vi "Example Threshold - CurrentReached Callback.vi"(4 "CurrentReached":refnum<user-event>, 5 "Event Data":T1, 6 "Control Ref":refnum<k24>, 7 "Event Common Data":T2) -> ()   [LabVIEW 2010]
uses:
  C:/tf/play/labview/Tinkerforge.dll
  Tinkerforge.dll
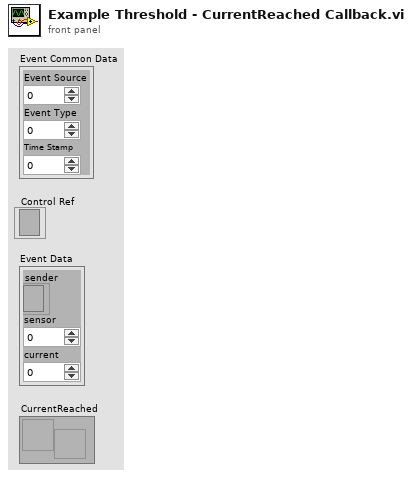
[diagram p1: front panel]
types:
  T1 = cluster{"sender":refnum<k24>, "sensor":u8, "current":i32}
  T2 = cluster{"Event Source":i32, "Event Type":u32, "Time Stamp":u32}
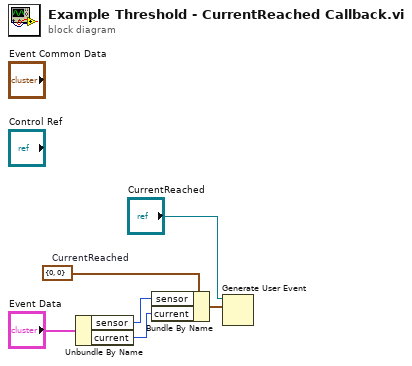
[diagram p0: block diagram]
diagram:
  w5 = cluster{"sensor":u8, "current":i32} {"sensor"=0, "current"=0}  # CurrentReached
  n1 = Unbundle By Name("Event Data") -> ("sensor"=w4:u8, "current"=w3:i32)
  n2 = Bundle By Name(cluster=w5, "sensor"=w4, "current"=w3) -> (w1:cluster{"sensor":u8, "current":i32})
  n3 = Generate User Event(user event="CurrentReached", event data cluster=w1) -> ()  [unwired: 1 in, 2 out]
